vi "Get DSF Version.vi"(8 "error in (no error)":errorcluster, 11 "configuration session in":refnum<class "Configuration Session.lvclass">) -> (0 "error out":errorcluster, 2 "dsf version":T1, 3 "configuration session out":refnum<class "Configuration Session.lvclass">)   [LabVIEW 2017, in "DSF Core.lvlib" / "Configuration Session.lvclass"]
doc: "Reads a value associated with a key in a specified section from the configuration data identified by <B>dsf refnum</B>. If the key does not exist, the VI returns the default value. This VI supports multibyte characters in strings. Wire data to the <B>default value</B> input to determine the polymorphic instance to use or manually select the instance."
uses:
  Configuration Session.lvclass
  Typedefs/DSF Version Info.ctl
  Configuration Session.lvclass/Configuration Session.ctl
  DSF Core.lvlib
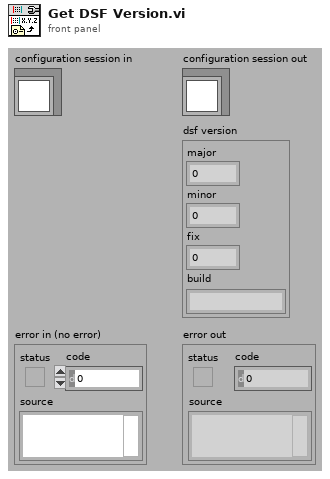
[diagram p1: front panel]
types:
  T1 = typedef "DSF Core.lvlib/DSF Version Info.ctl" = cluster{"major":u32, "minor":u32, "fix":u32, "build":string}
  T2 = typedef "DSF Core.lvlib/Configuration Session.lvclass/DSF Config Data Ref.ctl" = refnum<data-value>
  T3 = typedef "DSF Core.lvlib/Configuration Session.lvclass/DSF Config Data.ctl" = cluster{"dsf configuration":T4, "path":path, "dirty":bool}
  T4 = typedef "DSF Core.lvlib/Configuration Session.lvclass/Internal DSF Configuration.ctl" = cluster{"dsfversion":T1, "version":T1, "plugins":T5[], "groups":T10[], "transfers":T12[], "channels":T14[], "settings":T16[], "framework configuration":T18}
  T5 = typedef "DSF Core.lvlib/Configuration Session.lvclass/Internal DSF Plugin with ID.ctl" = cluster{"id":string, "values":T6}
  T6 = typedef "DSF Core.lvlib/Configuration Session.lvclass/Internal DSF Plugin Info.ctl" = cluster{"components":string[], "timing":T7, "group ids":string[], "settings id":string, "threads":T8[]}
  T7 = typedef "DSF Core.lvlib/DSF Timing Info.ctl" = cluster{"priority":u64, "decimation":u64, "offset":u64}
  T8 = typedef "DSF Core.lvlib/DSF Engine Plugin Thread Configuration.ctl" = cluster{"buffer converter settings":T9, "transceiver settings":T9, "custom settings":T9, "processor":i32, "priority offset":i16}
  T9 = typedef "DSF Core.lvlib/DSF Settings Info.ctl" = cluster{"key":string, "value":string}[]
  T10 = typedef "DSF Core.lvlib/Configuration Session.lvclass/Internal DSF Group with ID.ctl" = cluster{"id":string, "values":T11}
  T11 = typedef "DSF Core.lvlib/Configuration Session.lvclass/Internal DSF Group Info.ctl" = cluster{"direction":i32, "timing":T7, "transfer ids":string[], "settings id":string, "thread":i32, "timeout behavior":u8}
  T12 = typedef "DSF Core.lvlib/Configuration Session.lvclass/Internal DSF Transfer with ID.ctl" = cluster{"id":string, "values":T13}
  T13 = typedef "DSF Core.lvlib/Configuration Session.lvclass/Internal DSF Transfer Info.ctl" = cluster{"byte order":i32, "channel ids":string[], "settings id":string}
  T14 = typedef "DSF Core.lvlib/Configuration Session.lvclass/Internal DSF Channel with ID.ctl" = cluster{"id":string, "values":T15}
  T15 = typedef "DSF Core.lvlib/Configuration Session.lvclass/Internal DSF Channel Info.ctl" = cluster{"string buffer offset":u64, "string data type":i32, "engine data type":i32, "settings id":string, "units":string}
  T16 = typedef "DSF Core.lvlib/Configuration Session.lvclass/Internal DSF Settings with ID.ctl" = cluster{"id":string, "values":T17}
  T17 = typedef "DSF Core.lvlib/Configuration Session.lvclass/Internal DSF Settings Info.ctl" = cluster{"key":string, "value":string}[]
  T18 = typedef "DSF Core.lvlib/DSF Engine Framework Configuration.ctl" = cluster{"Plugins":T19[]}
  T19 = typedef "DSF Core.lvlib/DSF Engine Plugin Configuration.ctl" = cluster{"name":string, "components":string[], "cycle timing":T7, "threads":T8[], "Transfer Groups":T20[], "settings":T9}
  T20 = typedef "DSF Core.lvlib/DSF Engine Transfer Group Configuration.ctl" = cluster{"name":string, "direction":T21, "cycle timing":T7, "thread index":i32, "settings":T9, "Transfers":T22[], "timeout behavior":T26}
  T21 = typedef "DSF Core.lvlib/DSF Direction.ctl" = enum8{"Tx", "Rx"}
  T22 = typedef "DSF Core.lvlib/DSF Engine Transfer Configuration.ctl" = cluster{"name":string, "byte order":T23, "settings":T9, "channels":T24[]}
  T23 = typedef "DSF Core.lvlib/DSF Byte Order.ctl" = enum8{"big-endian", "little-endian"}
  T24 = typedef "DSF Core.lvlib/DSF Engine Channel Configuration.ctl" = cluster{"string offset":u64, "string data type":T25, "engine data type":T25, "name":string, "settings":T9, "units":string}
  T25 = typedef "DSF Core.lvlib/DSF Data Type.ctl" = enum8{"Bool", "SGL", "DBL", "I8", "I16", "I32", "I64", "U8", "U16", "U32", "U64"}
  T26 = typedef "DSF Core.lvlib/DSF Timeout Behavior.ctl" = enum8{"Increment Late Count", "Throw Error"}
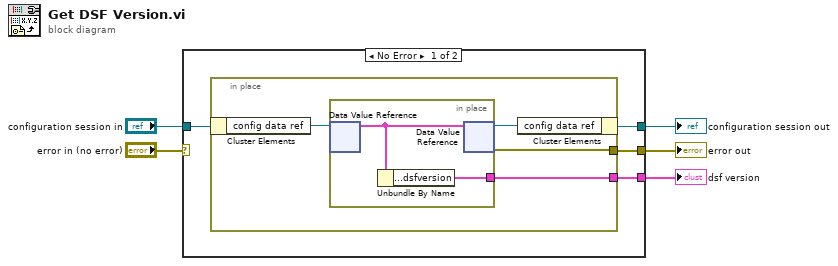
[diagram p0: block diagram]
diagram:
  n1 = case shown="No Error" "error in (no error)" {
    selector: "error in (no error)" -> [_ w17]
    tunnel: "configuration session in" -> [w8 w16]
    tunnel: [w9 w17] -> w4
    tunnel: [w7 w16] -> w1
    tunnel: [w6 _] -> w2
    frame No Error {
      n2 = in-place {
        in-place-border: [w13] -> w9
        in-place-border: [w10] -> w6
        n3 = in-place-cluster #1(w8) -> ("config data ref"=w11:T2)
        n4 = in-place {
          in-place-border: [w15] -> w10
          n5 = in-place-dvr #2(w11) -> (w14:T3)  [unwired: 1 out]
          n6 = Unbundle By Name(w14) -> ("dsf configuration.dsfversion"=w15:T1)
          n7 = in-place-dvr #2(w14) -> (w12:T2, w13:errorcluster)
        }
        n8 = in-place-cluster #1("config data ref"=w12) -> (w7:refnum<class "Configuration Session.lvclass">)
      }
    }
    frame Error {
    }
  }
  "error out" <- w4
  "configuration session out" <- w1
  "dsf version" <- w2
